vi "Load and Run.vi"(8 "error in (no error)":errorcluster, 10 "Subsystem URL":refnum<k21>, 11 "Subview":string) -> (0 "error out":errorcluster, 2 "Current Stop Event":refnum<user-event>, 3 "Subview VI Reference":refnum<vi>)   [LabVIEW 2024]
doc: "Loads the selected subview and runs the subview."
uses:
  Shared/User Event - Stop.lvlib
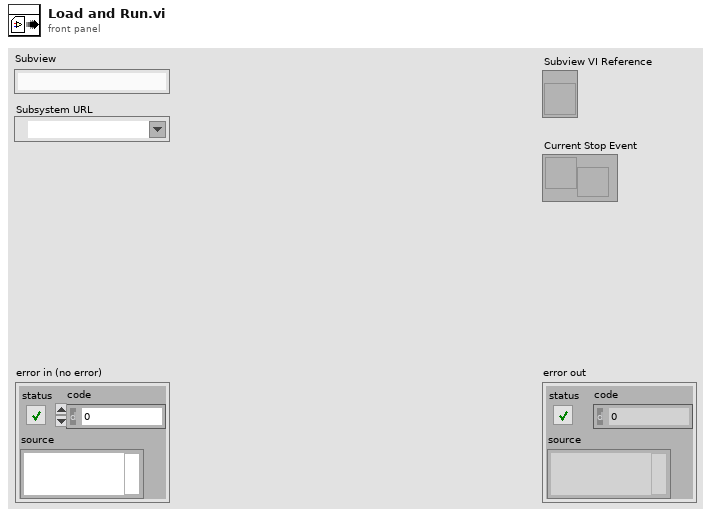
[diagram p1: front panel]
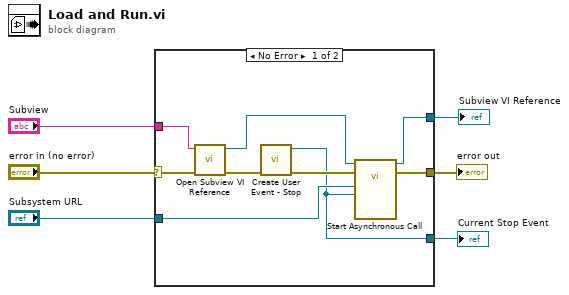
[diagram p0: block diagram]
diagram:
  n1 = case shown="No Error" "error in (no error)" {
    selector: "error in (no error)" -> [w10 w16]
    tunnel: [w14 _] -> w1
    tunnel: [w15 w16] -> w5
    tunnel: "Subview" -> [w9 _]
    tunnel: [w7 _] -> w3
    tunnel: "Subsystem URL" -> [w12 _]
    frame No Error {
      n2 = call "Open Subview VI Reference.vi"("error in (no error)"=w10, "Subview String"=w9) -> ("error out"=w11:errorcluster, "Subview VI Reference"=w8:refnum<vi>)  [unwired: 8 in]
      n3 = call "Create User Event - Stop.vi"("error in (no error)"=w11) -> ("error out"=w13:errorcluster, "User Event - Stop"=w7:refnum<user-event>)  [unwired: 9 in]
      n4 = call-by-ref "Start Asynchronous Call"(reference=w8, error in=w13, "Subview Stop Event"=w7, "Sub-system URL"=w12) -> (reference out=w14:refnum<vi>, error out=w15:errorcluster)  [unwired: 10 in]
    }
    frame Error {
    }
  }
  "error out" <- w5
  "Current Stop Event" <- w3
  "Subview VI Reference" <- w1
